vi "Display Units.vi"(8 "error in (no error)":errorcluster, 11 "VISA resource name":refnum<visa-resource-name>) -> (0 "error out":errorcluster, 2 "Units":string, 3 "VISA resource name out":refnum<visa-resource-name>)   [LabVIEW 2009, in "Newport 1830-C.lvlib"]
doc: "Reads units from instrument and ouputs symbol as a string."
uses:
  Newport 1830-C.lvlib
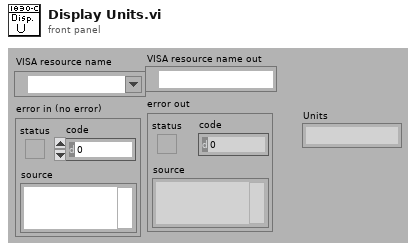
[diagram p1: front panel]
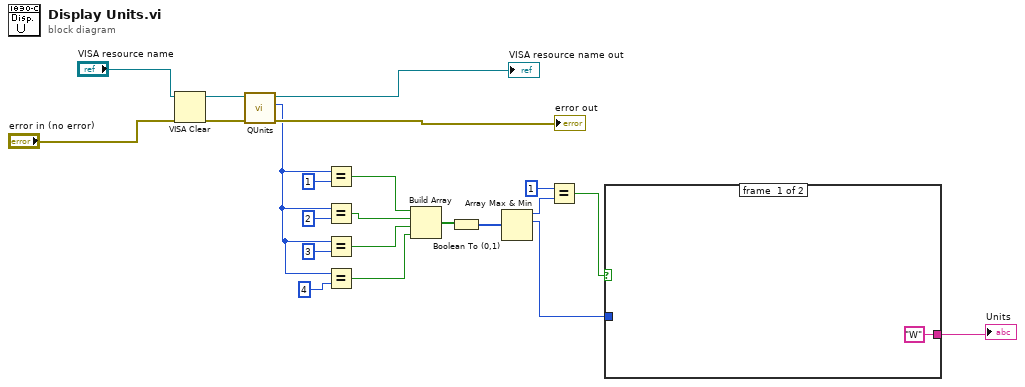
[diagram p0: block diagram]
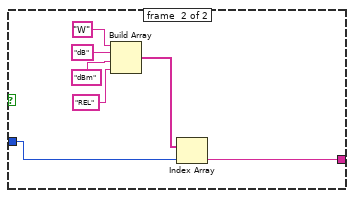
[diagram p2: hidden frame]
diagram:
  n1 = VISA Clear() -> ()  [unwired: 2 in, 2 out]
  n2 = call "QUnits.vi"("error in (no error)"="error in (no error)", "VISA resource name"="VISA resource name") -> ("error out"=→"error out":errorcluster, "Units"=w16:u32, "VISA resource name out"=→"VISA resource name out":refnum<visa-resource-name>)  [unwired: 6 in, 1 out]
  n3 = Equal?(x=w16, y=1) -> (x = y?=w11:bool)
  n4 = Equal?(x=w16, y=2) -> (x = y?=w10:bool)
  n5 = Equal?(x=w16, y=3) -> (x = y?=w9:bool)
  n6 = Equal?(x=w16, y=4) -> (x = y?=w8:bool)
  n7 = Build Array(w11, w10, w9, w8) -> (w7:bool[])
  n8 = Boolean To (0,1)(Boolean=w7) -> (0, 1=w6:i16[])
  n9 = Array Max & Min(array=w6) -> (max value=w3:i16, max index (indices)=w5:i32)  [unwired: 2 out]
  n10 = Equal?(x=i16 1, y=w3) -> (x = y?=w1:bool)
  n11 = case shown="True" w1 {
    tunnel: w5 -> [_ w23]
    tunnel: ["W" w22] -> w4
    frame #0 {
    }
    frame #1 {
      n12 = Build Array("W", "dB", "dBm", "REL") -> (w24:string[])
      n13 = Index Array(array=w24, index=w23) -> (element=w22:string)
    }
  }
  "Units" <- w4
